vi "Get Dev Par Info.vi"(10 "pstDevParInfo":T1, 11 "devId":i32) -> (1 "devId out":i32, 2 "pstDevParInfo out":T1, 3 "function return":i32)   [LabVIEW 2013, in "CHR34XXX.lvlib"]
doc: "DLL BOOL __stdcall CHR34XXX_OpenDev(IN int devId); DLL BOOL __stdcall CHR34XXX_OpenDevEx(OUT int *devId,IN BYTE busNo,IN BYTE DevNo,IN BYTE FuncNo); DLL BOOL __stdcall CHR34XXX_CloseDev(IN int devId); DLL BOOL __stdcall CHR34XXX_ResetDev(IN int devId); DLL BOOL __stdcall CHR34XXX_GetDevParInfo(IN int devId,OUT pCHR_DEVPARST pstDevParInfo);"
uses:
  CHR34XXX.lvlib
  CHR34XXX.dll
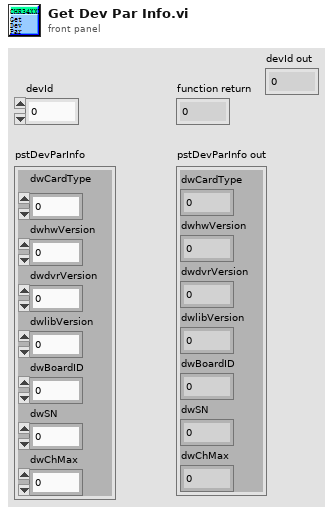
[diagram p1: front panel]
types:
  T1 = cluster{"dwCardType":u32, "dwhwVersion":u32, "dwdvrVersion":u32, "dwlibVersion":u32, "dwBoardID":u32, "dwSN":u32, "dwChMax":u32}
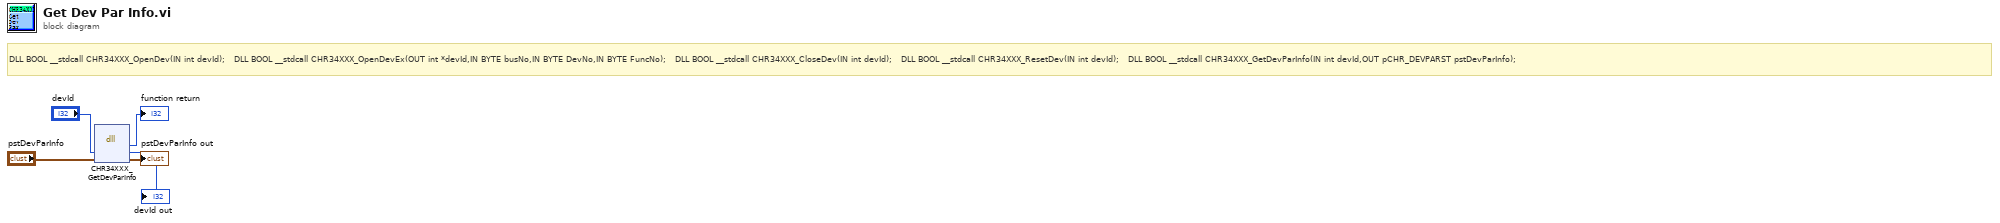
[diagram p0: block diagram]
diagram:
  # "DLL BOOL __stdcall CHR34XXX_OpenDev(IN int devId);   DLL BOOL __stdcall CHR34XXX_OpenDevEx(OUT int *devId,IN BYTE busNo,IN BYTE DevNo,IN BYTE FuncNo);   DLL BOOL __stdcall CHR34XXX_CloseDev(IN int devId);   DLL BOOL __stdcall CHR34XXX_ResetDev(IN int devId);   DLL BOOL __stdcall CHR34XXX_GetDevParInfo(IN int devId,OUT pCHR_DEVPARST pstDevParInfo);"
  n1 = dll-call lib="C:/Users/dy/Desktop/CHR34XXX_lv/lv_lib/CHR34XXX.*" fn="CHR34XXX_GetDevParInfo"("devId"="devId", "pstDevParInfo"="pstDevParInfo") -> ("返回类型"=→"function return":i32, "devId"=→"devId out":i32, "pstDevParInfo"=→"pstDevParInfo out":T1)  [unwired: 3 in, 2 out]
